vi "GetHelp.vi"(11 "BuildSolution in":refnum<class "BuildSolution.lvclass">) -> (2 "Help":string, 3 "BuildSolution out":refnum<class "BuildSolution.lvclass">)   [LabVIEW 2019, in "BuildSolution.lvclass"]
uses:
  BuildSolution.lvclass
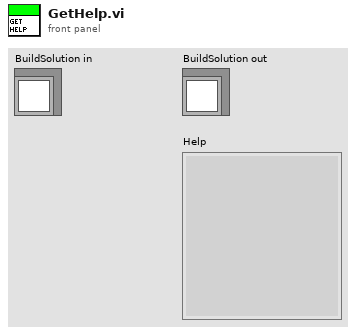
[diagram p1: front panel]
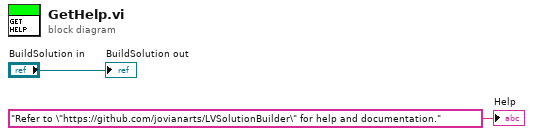
[diagram p0: block diagram]
diagram:
  "BuildSolution out" <- "BuildSolution in"
  "Help" <- "Refer to \"https://github.com/jovianarts/LVSolutionBuilder\" for help and documentation." ("Help")
